vi "output.vi"(8 "error in":errorcluster, 10 "data table in":T1, 11 "Scan Engine runtime in":refnum<class "Scan Engine runtime.lvclass">) -> (0 "error out":errorcluster, 2 "data table out":T1, 3 "Scan Engine runtime out":refnum<class "Scan Engine runtime.lvclass">)   [LabVIEW 2013, in "Scan Engine runtime.lvclass"]
doc: "Provides an interface for writing data to a module at runtime. While this interface performs no operations, a child should provide an override which may write to any open sessions, references, or interfaces."
uses:
  Scan Engine runtime.lvclass
  <vilib>/NI/Tag Bus/table/data table.ctl
  Scan Engine runtime.lvclass/Scan Engine runtime.ctl
  <vilib>/NI/Tag Bus/table/data polymorphs/read one/read Double.vi
  <vilib>/NI/Tag Bus/table/data polymorphs/read one/read Single.vi
  <vilib>/NI/Tag Bus/table/data polymorphs/read one/read I64.vi
  <vilib>/NI/Tag Bus/table/data polymorphs/read one/read I32.vi
  <vilib>/NI/Tag Bus/table/data polymorphs/read one/read I16.vi
  <vilib>/NI/Tag Bus/table/data polymorphs/read one/read I8.vi
  <vilib>/NI/Tag Bus/table/data polymorphs/read one/read U64.vi
  <vilib>/NI/Tag Bus/table/data polymorphs/read one/read U32.vi
  <vilib>/NI/Tag Bus/table/data polymorphs/read one/read U16.vi
  <vilib>/NI/Tag Bus/table/data polymorphs/read one/read U8.vi
  <vilib>/NI/Tag Bus/table/data polymorphs/read one/read Boolean.vi
  <vilib>/NI/Tag Bus/table/data table.lvlib
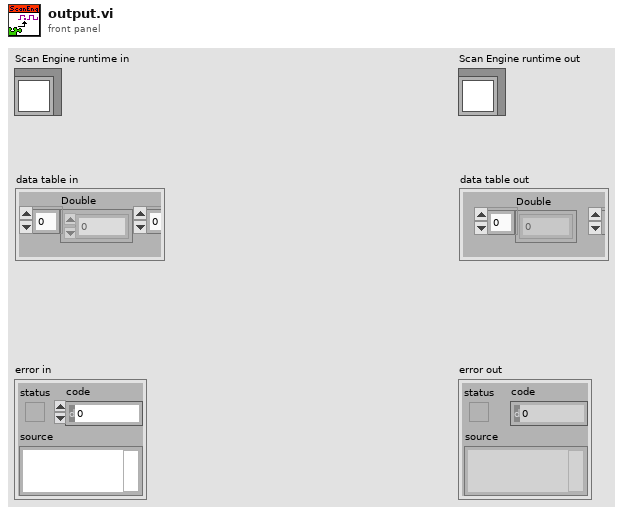
[diagram p1: front panel]
types:
  T1 = typedef "tag bus.lvlib/data table.lvlib/data table.ctl" = cluster{"Double":dbl[], "Single":sgl[], "I64":i64[], "I32":i32[], "I16":i16[], "I8":i8[], "U64":u64[], "U32":u32[], "U16":u16[], "U8":u8[], "Boolean":bool[], "String":string[], "Array of Double":cluster{"DBL Array":dbl[]}[], "Array of Single":cluster{"SGL Array":sgl[]}[], "Array of I64":cluster{"I64 Array":i64[]}[], "Array of I32":cluster{"I32 Array":i32[]}[], "Array of I16":cluster{"I16 Array":i16[]}[], "Array of I8":cluster{"I8 Array":i8[]}[], "Array of U64":cluster{"U64 Array":u64[]}[], "Array of U32":cluster{"U32 Array":u32[]}[], "Array of U16":cluster{"U16 Array":u16[]}[], "Array of U8":cluster{"U8 Array":u8[]}[], "Array of Boolean":cluster{"Boolean Array":bool[]}[], "Array of String":cluster{"String Array":string[]}[]}
  T2 = typedef "Scan Engine runtime.lvclass/Index Map.ctl" = cluster{"data type":T3, "variable ref":refnum<k21>, "index":i32}
  T3 = typedef "tag bus.lvlib/tag descriptor.lvclass/Data Type.ctl" = enum16{"Double", "Single", "I64", "I32", "I16", "I8", "U64", "U32", "U16", "U8", "Boolean", "String", "Array of Double", "Array of Single", "Array of I64", "Array of I32", "Array of I16", "Array of I8", "Array of U64", "Array of U32", "Array of U16", "Array of U8", "Array of Boolean", "Array of String"}
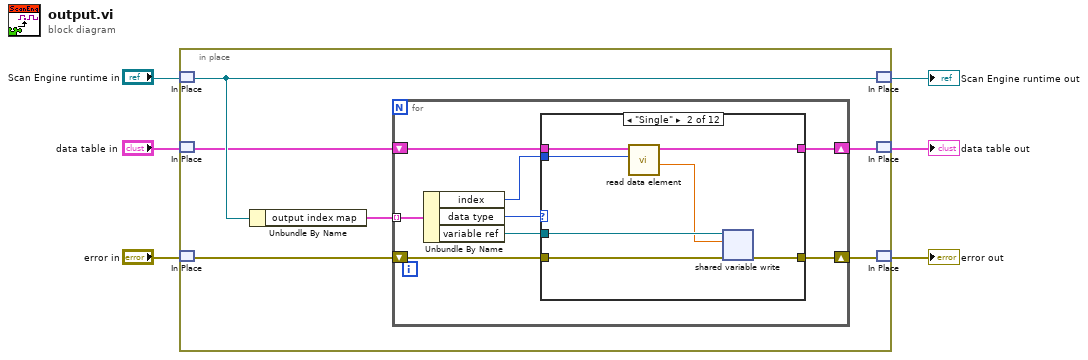
[diagram p0: block diagram]
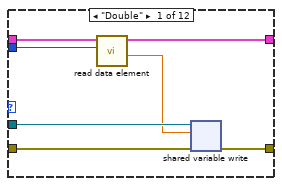
[diagram p2: hidden frame]
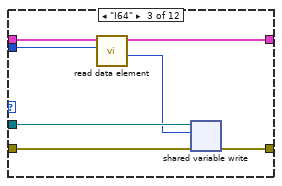
[diagram p3: hidden frame]
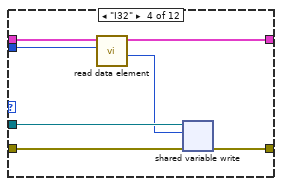
[diagram p4: hidden frame]
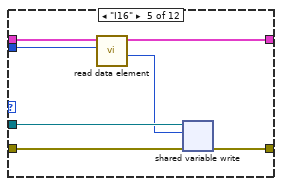
[diagram p5: hidden frame]
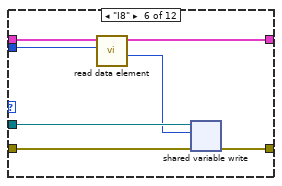
[diagram p6: hidden frame]
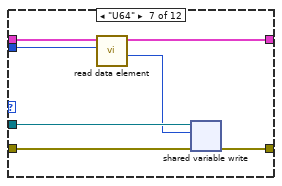
[diagram p7: hidden frame]
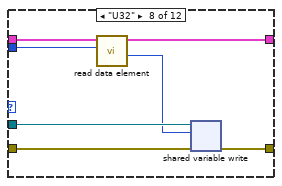
[diagram p8: hidden frame]
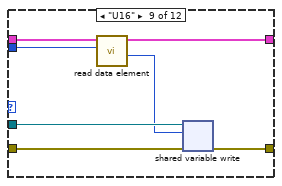
[diagram p9: hidden frame]
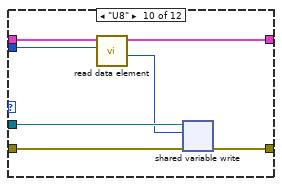
[diagram p10: hidden frame]
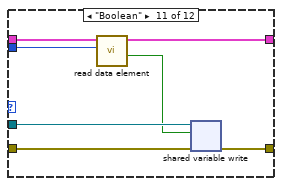
[diagram p11: hidden frame]
diagram:
  n1 = in-place {
    n2 = in-place-match #1("Scan Engine runtime in") -> (w12:refnum<class "Scan Engine runtime.lvclass">)
    n3 = in-place-match #2("data table in") -> (w11:T1)
    n4 = in-place-match #3("error in") -> (w8:errorcluster)
    n5 = Unbundle By Name(w12) -> ("output index map"=w9:T2[])
    n6 = for {
      shift-right: [w17] -> w10
      shift-left: w11 -> [w18]
      tunnel: w9 -> [w20] mode=indexing
      shift-right: [w14] -> w7
      shift-left: w8 -> [w16]
      n7 = Unbundle By Name(w20) -> ("index"=w13:i32, "data type"=w19:T3, "variable ref"=w15:refnum<k21>)
      n8 = case shown="\"Single\"" w19 {
        tunnel: w18 -> [w25 w32 w39 w46 w53 w60 w67 w74 w81 w88 w95 w99]
        tunnel: [w23 w30 w37 w44 w51 w58 w65 w72 w79 w86 w93 w99] -> w17
        tunnel: w16 -> [w26 w33 w40 w47 w54 w61 w68 w75 w82 w89 w96 w98]
        tunnel: w15 -> [w22 w29 w36 w43 w50 w57 w64 w71 w78 w85 w92 _]
        tunnel: [w27 w34 w41 w48 w55 w62 w69 w76 w83 w90 w97 w98] -> w14
        tunnel: w13 -> [w24 w31 w38 w45 w52 w59 w66 w73 w80 w87 w94 _]
        frame "Double" {
          n9 = call-poly <vilib>:"read data element.vi"("index"=w24, "data table in"=w25) -> ("value"=w21:dbl, "data table out"=w23:T1)  [unwired: 8 in]
          n10 = shared-variable-write(w22, w26, w21) -> (w27:errorcluster)  [unwired: 1 out]
        }
        frame "Single" {
          n11 = call-poly <vilib>:"read data element.vi"("index"=w31, "data table in"=w32) -> ("value"=w28:sgl, "data table out"=w30:T1)  [unwired: 8 in]
          n12 = shared-variable-write(w29, w33, w28) -> (w34:errorcluster)  [unwired: 1 out]
        }
        frame "I64" {
          n13 = call-poly <vilib>:"read data element.vi"("index"=w38, "data table in"=w39) -> ("value"=w35:i64, "data table out"=w37:T1)  [unwired: 8 in]
          n14 = shared-variable-write(w36, w40, w35) -> (w41:errorcluster)  [unwired: 1 out]
        }
        frame "I32" {
          n15 = call-poly <vilib>:"read data element.vi"("index"=w45, "data table in"=w46) -> ("value"=w42:i32, "data table out"=w44:T1)  [unwired: 8 in]
          n16 = shared-variable-write(w43, w47, w42) -> (w48:errorcluster)  [unwired: 1 out]
        }
        frame "I16" {
          n17 = call-poly <vilib>:"read data element.vi"("index"=w52, "data table in"=w53) -> ("value"=w49:i16, "data table out"=w51:T1)  [unwired: 8 in]
          n18 = shared-variable-write(w50, w54, w49) -> (w55:errorcluster)  [unwired: 1 out]
        }
        frame "I8" {
          n19 = call-poly <vilib>:"read data element.vi"("index"=w59, "data table in"=w60) -> ("value"=w56:i8, "data table out"=w58:T1)  [unwired: 8 in]
          n20 = shared-variable-write(w57, w61, w56) -> (w62:errorcluster)  [unwired: 1 out]
        }
        frame "U64" {
          n21 = call-poly <vilib>:"read data element.vi"("index"=w66, "data table in"=w67) -> ("value"=w63:u64, "data table out"=w65:T1)  [unwired: 8 in]
          n22 = shared-variable-write(w64, w68, w63) -> (w69:errorcluster)  [unwired: 1 out]
        }
        frame "U32" {
          n23 = call-poly <vilib>:"read data element.vi"("index"=w73, "data table in"=w74) -> ("value"=w70:u32, "data table out"=w72:T1)  [unwired: 8 in]
          n24 = shared-variable-write(w71, w75, w70) -> (w76:errorcluster)  [unwired: 1 out]
        }
        frame "U16" {
          n25 = call-poly <vilib>:"read data element.vi"("index"=w80, "data table in"=w81) -> ("value"=w77:u16, "data table out"=w79:T1)  [unwired: 8 in]
          n26 = shared-variable-write(w78, w82, w77) -> (w83:errorcluster)  [unwired: 1 out]
        }
        frame "U8" {
          n27 = call-poly <vilib>:"read data element.vi"("index"=w87, "data table in"=w88) -> ("value"=w84:u8, "data table out"=w86:T1)  [unwired: 8 in]
          n28 = shared-variable-write(w85, w89, w84) -> (w90:errorcluster)  [unwired: 1 out]
        }
        frame "Boolean" {
          n29 = call-poly <vilib>:"read data element.vi"("index"=w94, "data table in"=w95) -> ("value"=w91:bool, "data table out"=w93:T1)  [unwired: 8 in]
          n30 = shared-variable-write(w92, w96, w91) -> (w97:errorcluster)  [unwired: 1 out]
        }
        frame Default {
        }
      }
    }
    n31 = in-place-match #1(w12) -> (→"Scan Engine runtime out":refnum<class "Scan Engine runtime.lvclass">)
    n32 = in-place-match #2(w10) -> (→"data table out":T1)
    n33 = in-place-match #3(w7) -> (→"error out":errorcluster)
  }
